vi "iccid_PCAN.vi"(11 "iccid data":u8[][](array[numeric]) format="%.0x") -> (3 "iccid":string)   [LabVIEW 2024, in "PCANusb_DTU.lvlib"]
uses:
  PCANusb_DTU.lvlib
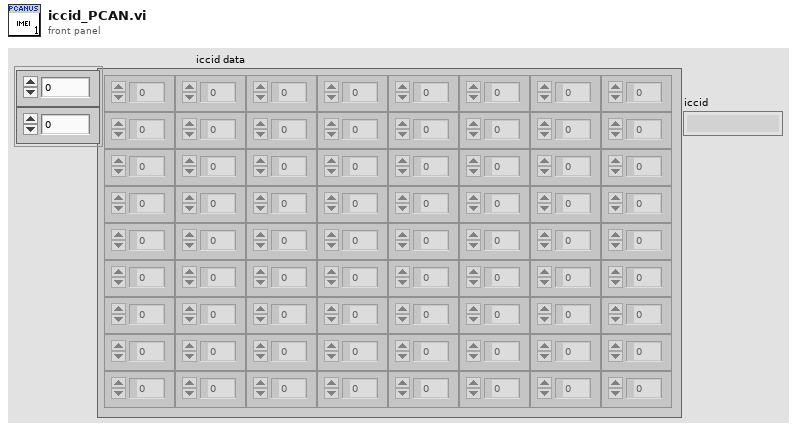
[diagram p1: front panel]
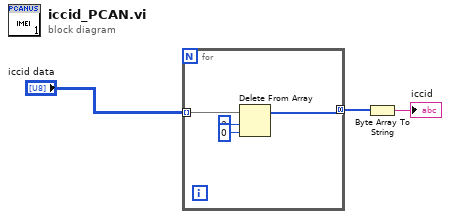
[diagram p0: block diagram]
diagram:
  n1 = for {
    tunnel: "iccid data" -> [w7] mode=indexing
    tunnel: [w4] -> w3 mode=concatenating
    n2 = Delete From Array(array=w7, length=3, index=0) -> (array with subset deleted=w4:u8[])  [unwired: 1 out]
  }
  n3 = Byte Array To String(unsigned byte array=w3) -> (string=→"iccid":string)
